vi "Save_Ensight.vi"() -> (5 "Plug in titles":string[](array[string]), 7 "Plug in values":string[](array[string]))   [LabVIEW 2011]
uses:
  Globals/Plug_in_data_global.vi
  Globals/LDA_meas_global_1.vi
  Globals/Meas_global.vi
  Globals/Constants_global.vi
  <vilib>/ptbypt/NI_PtbyPt.lvlib
panel:
  out "Temp File Path":path
  out "concatenated string":string
  out "Results Array":string[](array[string])
  out "IJ Values":i32[](array[numeric])
  out "Latest Data":dbl[][](array[numeric])
  out "Variables":dbl[][](array[numeric])
  out "Results File Path":path
  out "Processing first block?":bool
  out "XY Position":string[](array[string])
  out "Results File Exists?":bool
  # "You must have just these two indicators on the connector pane of the vi"
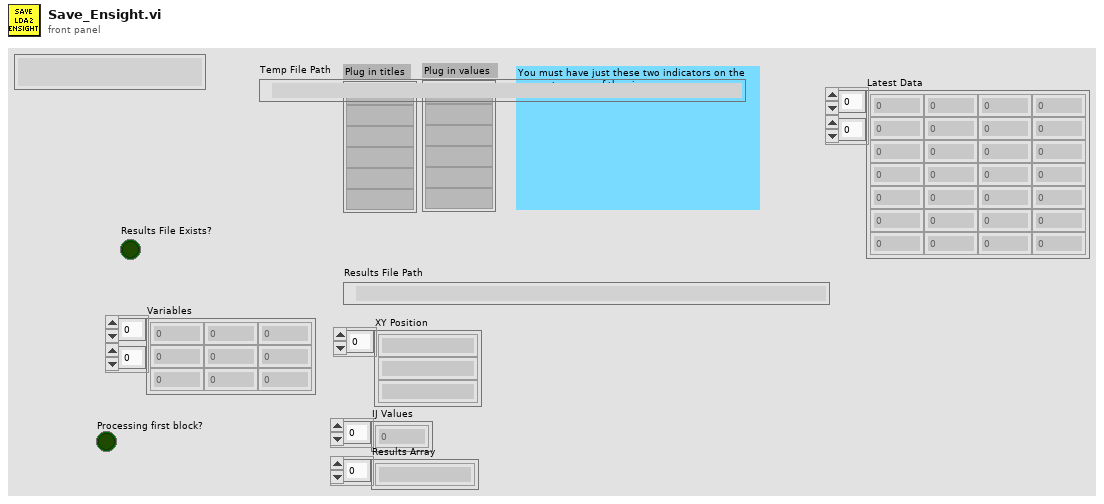
[diagram p1: front panel]
types:
  T1 = typedef "Analysis_info_cluster.ctl" = cluster{"Colour":u32, "Inst type":T2, "Inst name":string, "Symbol":string, "Code name":string, "Extra Info":string, "Inst Array":T3, "Index":i32, "Voltage Index":i32, "Extra Titles":string[], "Extra Values":string[], "Eng Values":dbl[], "Time (ms)":dbl[], "Voltage":dbl[], "U":dbl, "u^2":dbl, "u^3":dbl, "u^4":dbl, "Skew_u":dbl, "Kurt_u":dbl, "Sd Error in Mean":dbl, "% u'/U":dbl, "X":dbl, "Y":dbl, "Z":dbl, "Spectra":T4, "Autocorrelation":T4, "Timescale integral to 25%":dbl, "Sd Error in Variance":dbl, "Calib File":path, "Calib Constants":dbl[], "Histogram":T4, "Output Position":bool, "Full Stats":bool, "Weighting":dbl[]}
  T2 = typedef "Inst_type.ctl" = enum16{"Propeller anemometer", "Raw voltage", "Pressure Transducer", "Pitot-static tube", "Preston tube", "Hot wire", "Cross wire 1", "Cross wire 2", "Generic Linear", "Generic Polynomial", "Generic BackPoly", "Fast FID", "Thermocouple", "Cold wire", "Pulsed Wire", "LDA Vel", "LDA Tran time", "LDA Arr time"}
  T3 = typedef "Instrument_Array.ctl" = enum16{"PWA", "LDA", "Analogue"}
  T4 = typedef "XY_Plot_Cluster.ctl" = cluster{"First Name":string, "Second Name":string, "X axis name":string, "Y axis name":string, "X array":dbl[], "Y array":dbl[]}
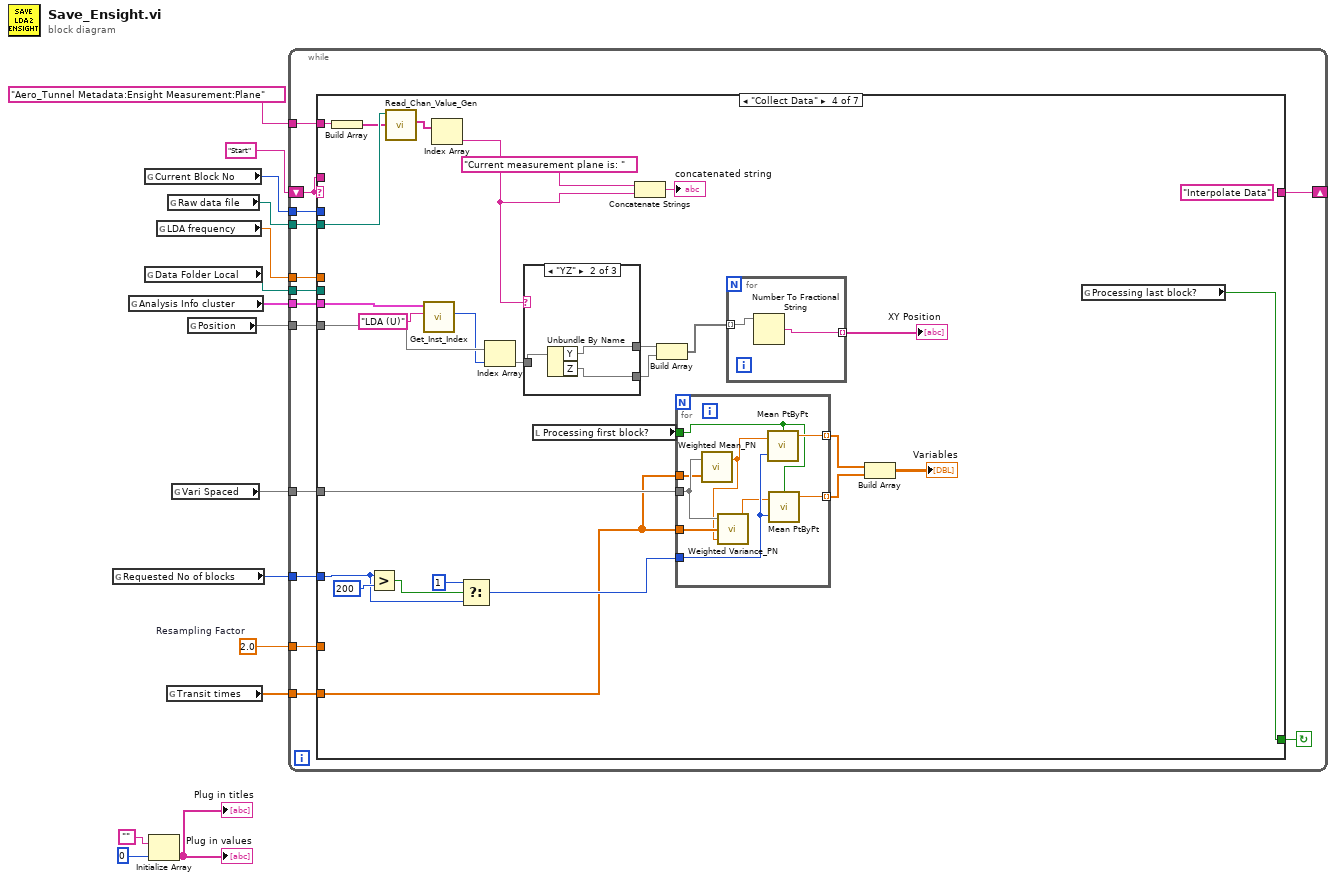
[diagram p0: block diagram]
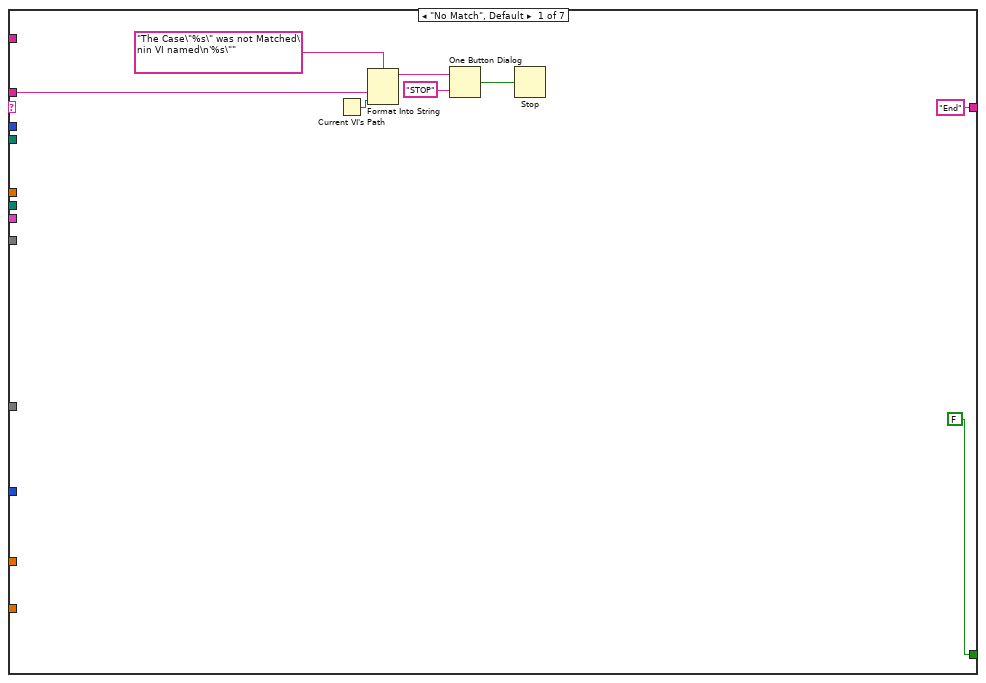
[diagram p2: hidden frame]
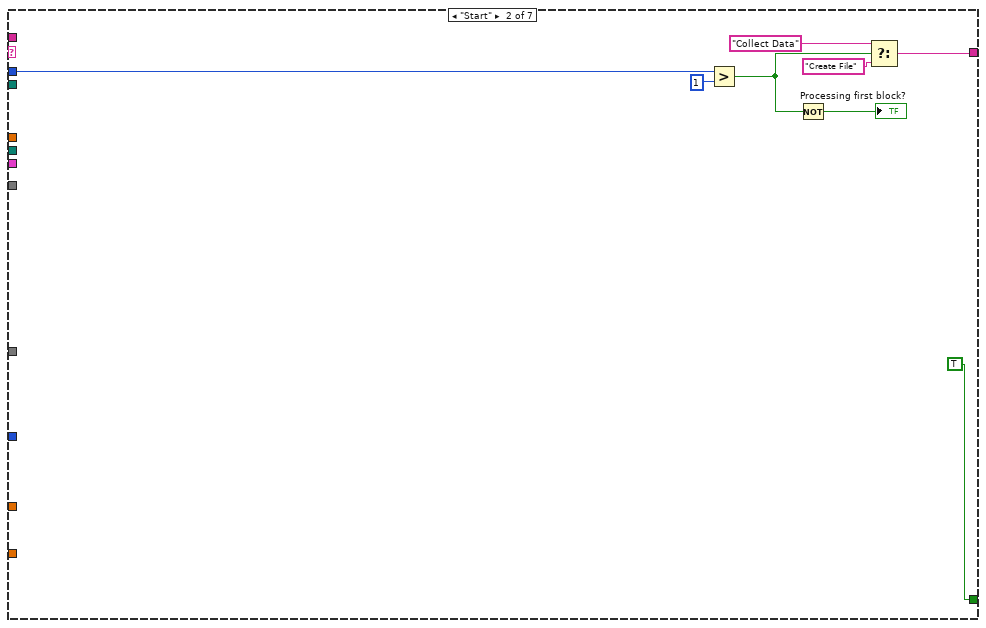
[diagram p3: hidden frame]
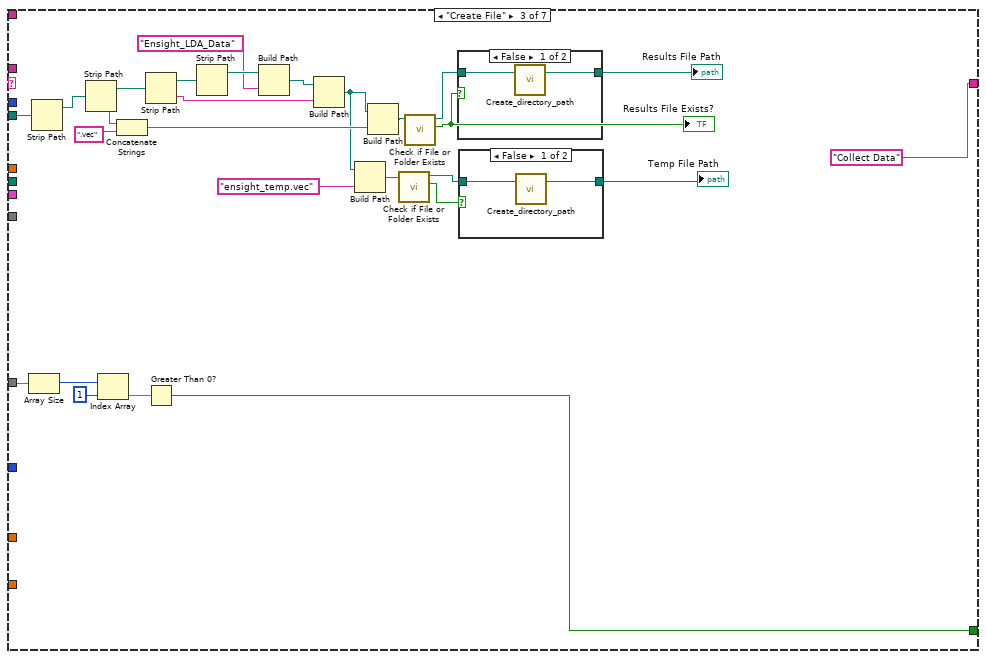
[diagram p4: hidden frame]
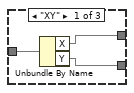
[diagram p7: hidden frame]
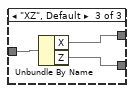
[diagram p8: hidden frame]
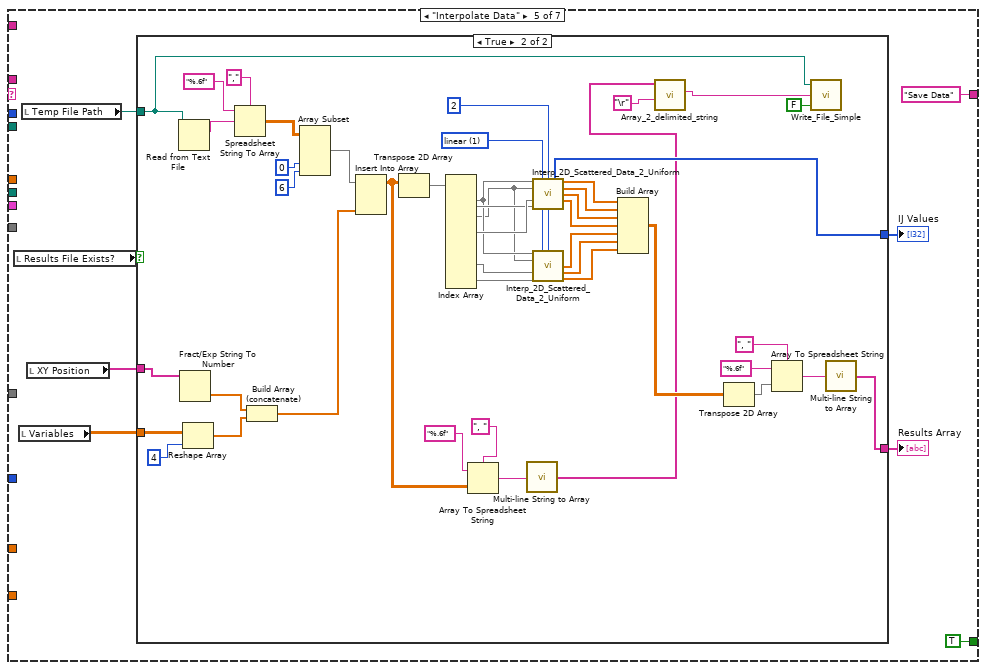
[diagram p9: hidden frame]
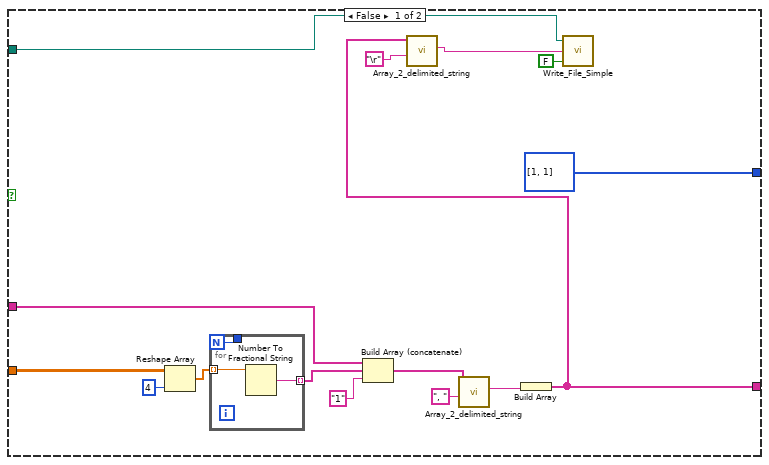
[diagram p10: hidden frame]
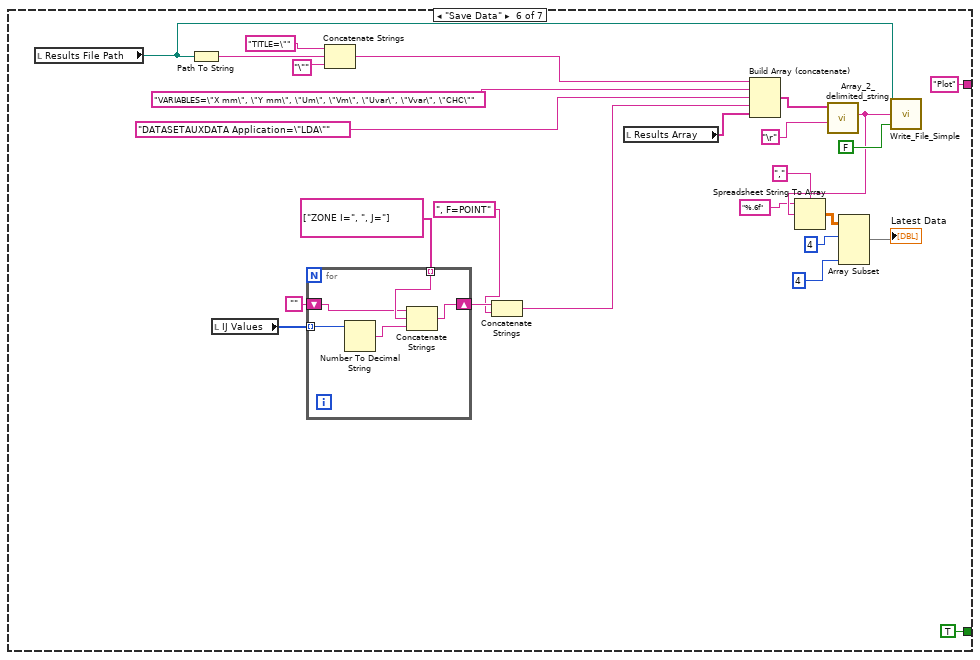
[diagram p11: hidden frame]
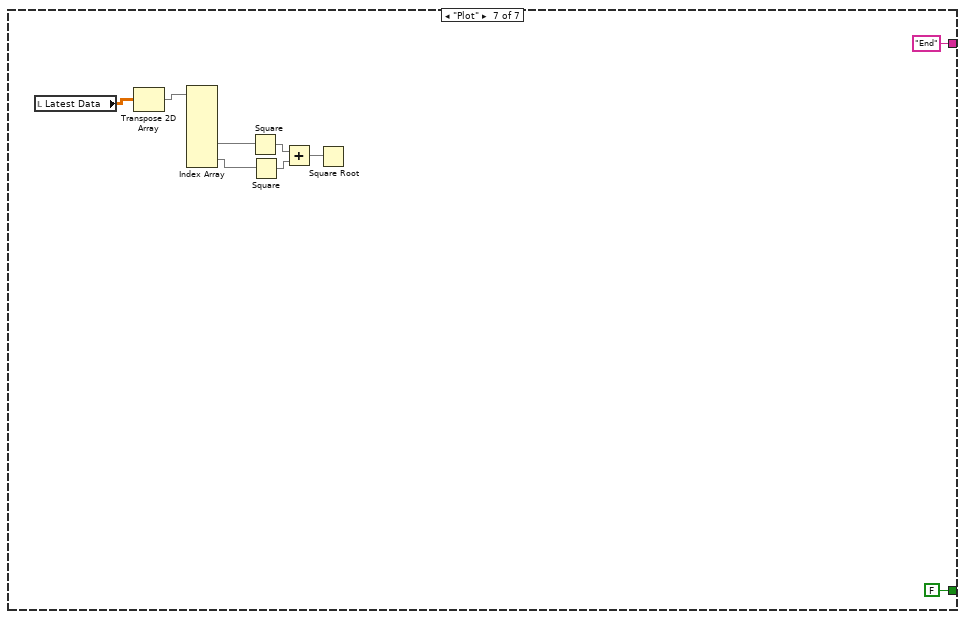
[diagram p12: hidden frame]
diagram:
  w6 = 2.0  # Resampling Factor
  n1 = global read "Meas_global.vi" "Requested No of blocks"() -> (w3:i32)
  n2 = global read "Meas_global.vi" "Analysis Info cluster"() -> (w4:T1[])
  n3 = global read "Meas_global.vi" "Current Block No"() -> (w9:i32)
  n4 = global read "Constants_global.vi" "Data Folder Local"() -> (w5:path)
  n5 = Initialize Array("", 0) -> (→"Plug in values" →"Plug in titles":string[])
  n6 = global read "Meas_global.vi" "LDA frequency"() -> (w7:dbl)
  n7 = global read "LDA_meas_global_1.vi" "Transit times"() -> (w13:dbl[])
  n8 = global read "Meas_global.vi" "Raw data file"() -> (w8:path)
  n9 = global read "Plug_in_data_global.vi" "Vari Spaced"() -> (w14)
  n10 = global read "Meas_global.vi" "Position"() -> (w2)
  n11 = while {
    shift-left: "Start" -> [w29]
    shift-right: [w26] -> _
    tunnel: w14 -> [w28]
    tunnel: w13 -> [w27]
    tunnel: w9 -> [w24]
    tunnel: w5 -> [w23]
    tunnel: w8 -> [w22]
    tunnel: w7 -> [w21]
    tunnel: w6 -> [w20]
    tunnel: w4 -> [w19]
    tunnel: w3 -> [w18]
    tunnel: w2 -> [w17]
    tunnel: "Aero_Tunnel Metadata:Ensight Measurement:Plane" -> [w16]
    stop <- w25 continue-if-true
    n12 = case shown="\"Collect Data\"" w29 {
      tunnel: ["End" ("t") w40 "Collect Data" ("t") "Interpolate Data" ("t") "Save Data" ("t") "Plot" ("t") "End" ("t")] -> w26
      tunnel: w29 -> [w33 _ _ _ _ _ _]
      tunnel: w28 -> [_ _ w71 w106 _ _ _]
      tunnel: w27 -> [_ _ _ w99 _ _ _]
      tunnel: [FALSE TRUE w67 w86 TRUE ("Processing last block?") TRUE ("Processing last block?") FALSE ("Processing last block?")] -> w25
      tunnel: w24 -> [_ w39 _ _ _ _ _]
      tunnel: w23 -> [_ _ _ _ _ _ _]
      tunnel: w22 -> [_ _ w66 w85 _ _ _]
      tunnel: w21 -> [_ _ _ _ _ _ _]
      tunnel: w20 -> [_ _ _ _ _ _ _]
      tunnel: w19 -> [_ _ _ w96 _ _ _]
      tunnel: w18 -> [_ _ _ w101 _ _ _]
      tunnel: w17 -> [_ _ _ w98 _ _ _]
      tunnel: w16 -> [_ _ _ w84 _ _ _]
      frame "No Match", Default {
        n13 = Current VI's Path() -> (path=w32:path)
        n14 = Format Into String(format string="The Case\"%s\" was not Matched\nin VI named\n'%s\"" ("Format String"), w33, w32) -> (resulting string=w36:string)  [unwired: 2 in, 1 out]
        n15 = One Button Dialog(message=w36, button name ("OK")="STOP") -> (true=w34:bool)
        n16 = Stop(stop? (T)=w34) -> ()
      }
      frame "Start" {
        n17 = Greater?(x=w39, y=1) -> (0:w42:bool)
        n18 = Not(x=w42) -> (.not. x?=→"Processing first block?":bool)
        n19 = Select(t="Collect Data", s=w42, f="Create File") -> (s? t:f=w40:string)
      }
      frame "Create File" {
        n20 = Array Size(array=w71) -> (size(s)=w70:i32)
        n21 = Strip Path(path=w66) -> (stripped path=w65:path)  [unwired: 1 out]
        n22 = Strip Path(path=w65) -> (stripped path=w64:path, name=w53:string)
        n23 = Index Array(array=w70, index=1) -> (element=w68)
        n24 = Concatenate Strings(w53, ".vec" ("string")) -> (w57:string)
        n25 = Strip Path(path=w64) -> (stripped path=w63:path, name=w59:string)
        n26 = Greater Than 0?(x=w68) -> (x > 0?=w67:bool)
        n27 = Strip Path(path=w63) -> (stripped path=w62:path)  [unwired: 1 out]
        n28 = Build Path(base path=w62, name or relative path="Ensight_LDA_Data") -> (appended path=w60:path)
        n29 = Build Path(base path=w60, name or relative path=w59) -> (appended path=w49:path)
        n30 = Build Path(base path=w49, name or relative path="ensight_temp.vec" ("string")) -> (appended path=w51:path)
        n31 = Build Path(base path=w49, name or relative path=w57) -> (appended path=w52:path)
        n32 = call <vilib>:"Check if File or Folder Exists.vi"("path"=w51) -> ("file or folder exists?"=w48:bool, "dup path"=w47:path)  [unwired: 8 in, 1 out]
        n33 = call <vilib>:"Check if File or Folder Exists.vi"("path"=w52) -> ("file or folder exists?"=w54:bool, "dup path"=w56:path)  [unwired: 8 in, 1 out]
        "Results File Exists?" <- w54
        n34 = case shown="False" w54 {
          tunnel: w56 -> [w77 w78]
          tunnel: [w76 w78] -> w55
          frame False {
            n35 = call "Create_directory_path.vi"("Path name"=w77) -> ("Path name Out"=w76:path)  [unwired: 1 in, 1 out]
          }
          frame True {
          }
        }
        "Results File Path" <- w55
        n36 = case shown="False" w48 {
          tunnel: w47 -> [w74 w75]
          tunnel: [w73 w75] -> w46
          frame False {
            n37 = call "Create_directory_path.vi"("Path name"=w74) -> ("Path name Out"=w73:path)  [unwired: 1 in, 1 out]
          }
          frame True {
          }
        }
        "Temp File Path" <- w46
      }
      frame "Collect Data" {
        n38 = Build Array(w84) -> (w83:string[])
        n39 = Greater?(x=w101, y=200) -> (0:w103:bool)
        n40 = call "Read_Chan_Value_Gen.vi"("Desired Ch Names"=w83, "Raw data file"=w85) -> ("Values"=w82:string[])  [unwired: 9 in]
        n41 = call "Get_Inst_Index.vi"("Inst name search"="LDA (U)", 11:w96) -> ("Index of Instance"=w95:i32)  [unwired: 7 in, 2 out]
        n42 = Index Array(array=w82) -> (element=w81:string)  [unwired: 1 in]
        n43 = Select(t=1, s=w103, f=w101) -> (s? t:f=w100:i32)
        n44 = Index Array(array=w98, index=w95) -> (element=w94)
        n45 = case shown="\"YZ\"" w81 {
          tunnel: w94 -> [w110 w113 w116]
          tunnel: [w109 w112 w115] -> w93
          tunnel: [w108 w111 w114] -> w92
          frame "XY" {
            n46 = Unbundle By Name(w110) -> ("X"=w109, "Y"=w108)
          }
          frame "YZ" {
            n47 = Unbundle By Name(w113) -> ("Y"=w112, "Z"=w111)
          }
          frame "XZ", Default {
            n48 = Unbundle By Name(w116) -> ("X"=w115, "Z"=w114)
          }
        }
        n49 = local read "Processing first block?"() -> (w105:bool)
        n50 = Concatenate Strings("Current measurement plane is: " ("string"), w81) -> (→"concatenated string":string)
        n51 = Build Array(w93, w92) -> (w88:void[])
        n52 = for {
          tunnel: w106 -> [w123]
          tunnel: [w127] -> w91 mode=indexing
          tunnel: [w126] -> w90 mode=indexing
          tunnel: w105 -> [w124]
          tunnel: w100 -> [w125]
          tunnel: w99 -> [w122]
          tunnel: w99 -> [w121]
          n53 = call "Weighted Mean_PN.vi"("weights"=w121, "1D data"=w123) -> ("Weighted mean"=w120:dbl)  [unwired: 1 in]
          n54 = call "Weighted Variance_PN.vi"("Weighted mean"=w120, "weights"=w122, "1D data"=w123) -> ("Weighted variance"=w119:dbl)  [unwired: 1 in]
          n55 = call <vilib>:"Mean PtByPt.vi"("x"=w120, "sample length"=w125, "initialize"=w124) -> ("mean"=w127:dbl)  [unwired: 1 in, 1 out]
          n56 = call <vilib>:"Mean PtByPt.vi"("x"=w119, "sample length"=w125, "initialize"=w124) -> ("mean"=w126:dbl)  [unwired: 1 in, 1 out]
        }
        n57 = for {
          tunnel: w88 -> [w118] mode=indexing
          tunnel: [w117] -> w87 mode=indexing
          n58 = Number To Fractional String(number=w118) -> (F-format string=w117:string)  [unwired: 3 in]
        }
        "XY Position" <- w87
        n59 = Build Array(w91, w90) -> (→"Variables":dbl[][])
        n60 = global read "Meas_global.vi" "Processing last block?"() -> (w86:bool)
      }
      frame "Interpolate Data" {
        n61 = local read "Results File Exists?"() -> (w131:bool)
        n62 = local read "Variables"() -> (w133:dbl[][])
        n63 = local read "Temp File Path"() -> (w128:path)
        n64 = local read "XY Position"() -> (w132:string[])
        n65 = case shown="True" w131 {
          tunnel: w133 -> [w150 w191]
          tunnel: [w139 w166] -> w129
          tunnel: w132 -> [w144 w192]
          tunnel: [i32[] [1, 1] w179] -> w130
          tunnel: w128 -> [w136 w162]
          frame False {
            n66 = Reshape Array(w150, 4 ("dimension size")) -> (w148:dbl[])
            n67 = for {
              N -> [w151]
              tunnel: w148 -> [w153] mode=indexing
              tunnel: [w152] -> w145 mode=indexing
              tunnel: [w151] -> _
              n68 = Number To Fractional String(number=w153) -> (F-format string=w152:string)  [unwired: 3 in]
            }
            n69 = Build Array (concatenate)(w144, w145, "1") -> (w143:string[])
            n70 = call "Array_2_delimited_string.vi"("delimiter (Tab)"=", ", "Array of Strings"=w143) -> ("delimited string"=w146:string)  [unwired: 9 in]
            n71 = Build Array(w146) -> (w139:string[])
            n72 = call "Array_2_delimited_string.vi"("delimiter (Tab)"="\r", "Array of Strings"=w139) -> ("delimited string"=w138:string)  [unwired: 9 in]
            n73 = call "Write_File_Simple.vi"("append to file? (new file:F)"=FALSE, "character string"=w138, "file path"=w136) -> ()  [unwired: 2 out]
          }
          frame True {
            w177 = 2 ("Interpolation Factor")
            w178 = 1 items=["nearest", "linear", "cubic", "biharmonic spline "] ("method")
            n74 = Read from Text File(file (use dialog)=w162) -> (text=w194:string)  [unwired: 3 in, 3 out]
            n75 = Fract/Exp String To Number(string=w192) -> (number=w189:dbl[])  [unwired: 3 in, 1 out]
            n76 = Reshape Array(w191, 4 ("index")) -> (w188:dbl[])
            n77 = Spreadsheet String To Array(delimiter (Tab)=",", format string="%.6f", spreadsheet string=w194) -> (array=w193:dbl[][])  [unwired: 1 in]
            n78 = Build Array (concatenate)(w189, w188) -> (w186:dbl[])
            n79 = Array Subset(array=w193, index (col)=0 ("index"), length (col)=6 ("length")) -> (w187:dbl[][])  [unwired: 2 in]
            n80 = Insert Into Array(array=w187, new element=w186) -> (w156:dbl[][])  [unwired: 2 in]
            n81 = Transpose 2D Array(2D array=w156) -> (transposed array=w185:dbl[][])
            n82 = Index Array(array=w185) -> (element #1=w182:dbl[], element #2=w154:dbl[], element #3=w184:dbl[], element #4=w183:dbl[], element #5=w181:dbl[], element #6=w180:dbl[])  [unwired: 12 in]
            n83 = Array To Spreadsheet String(delimiter (Tab)=", ", array=w156, 3:"%.6f" ("format string")) -> (spreadsheet string=w161:string)
            n84 = call "Multi-line String to Array.vi"("Multi lined string"=w161) -> ("Array of string lines"=w155:string[])
            n85 = call "Interp_2D_Scattered_Data_2_Uniform.vi"("X"=w182, "method"=w178, "Interpolation Factor"=w177, "Y"=w154, "U"=w184, "V"=w183) -> ("IJ Values"=w179:i32[], "Xi"=w176:dbl[], "Yi"=w175:dbl[], "Ui"=w174:dbl[], "Vi"=w173:dbl[])  [unwired: 4 in, 1 out]
            n86 = call "Interp_2D_Scattered_Data_2_Uniform.vi"("X"=w182, "method"=w178, "Interpolation Factor"=w177, "Y"=w154, "U"=w181, "V"=w180) -> ("Ui"=w172:dbl[], "Vi"=w171:dbl[], "Convex Hull Check"=w170:dbl[])  [unwired: 4 in, 3 out]
            n87 = Build Array(w176, w175, w174, w173, w172, w171, w170) -> (w168:dbl[][])
            n88 = call "Array_2_delimited_string.vi"("delimiter (Tab)"="\r", "Array of Strings"=w155) -> ("delimited string"=w164:string)  [unwired: 9 in]
            n89 = Transpose 2D Array(2D array=w168) -> (transposed array=w169:dbl[][])
            n90 = Array To Spreadsheet String(delimiter (Tab)=", ", array=w169, 3:"%.6f" ("format string")) -> (spreadsheet string=w167:string)
            n91 = call "Write_File_Simple.vi"("append to file? (new file:F)"=FALSE, "character string"=w164, "file path"=w162) -> ()  [unwired: 2 out]
            n92 = call "Multi-line String to Array.vi"("Multi lined string"=w167) -> ("Array of string lines"=w166:string[])
          }
        }
        "IJ Values" <- w130
        "Results Array" <- w129
      }
      frame "Save Data" {
        n93 = local read "Results File Path"() -> (w208:path)
        n94 = Path To String(path=w208) -> (string=w221:string)
        n95 = local read "IJ Values"() -> (w201:i32[])
        n96 = for {
          tunnel: w201 -> [w229] mode=indexing
          shift-right: [w227] -> w204
          shift-left: "" -> [w225]
          tunnel: string[] ["ZONE I=", ", J="] -> [w226] mode=indexing
          n97 = Number To Decimal String(number=w229) -> (decimal integer string=w228:string)  [unwired: 1 in]
          n98 = Concatenate Strings(w225, w226, w228) -> (w227:string)
        }
        n99 = Concatenate Strings("TITLE=\"" ("string"), w221, "\"" ("string")) -> (w219:string)
        n100 = Concatenate Strings(w204, ", F=POINT") -> (w202:string)
        n101 = local read "Results Array"() -> (w200:string[])
        n102 = Build Array (concatenate)(w219, "VARIABLES=\"X mm\", \"Y mm\", \"Um\", \"Vm\", \"Uvar\", \"Vvar\", \"CHC\"" ("string"), "DATASETAUXDATA Application=\"LDA\"", w202, w200) -> (w216:string[])
        n103 = call "Array_2_delimited_string.vi"("delimiter (Tab)"="\r", "Array of Strings"=w216) -> ("delimited string"=w214:string)  [unwired: 9 in]
        n104 = Spreadsheet String To Array(delimiter (Tab)=",", format string="%.6f", spreadsheet string=w214) -> (array=w213:dbl[][])  [unwired: 1 in]
        n105 = Array Subset(array=w213, index (row)=4 ("index"), length (col)=4 ("length")) -> (→"Latest Data":dbl[][])  [unwired: 2 in]
        n106 = call "Write_File_Simple.vi"("append to file? (new file:F)"=FALSE, "character string"=w214, "file path"=w208) -> ()  [unwired: 2 out]
      }
      frame "Plot" {
        n107 = local read "Latest Data"() -> (w236:dbl[][])
        n108 = Transpose 2D Array(2D array=w236) -> (transposed array=w235:dbl[][])
        n109 = Index Array(array=w235) -> (element #3=w234:dbl[], element #4=w233:dbl[])  [unwired: 8 in, 2 out]
        n110 = Square(x=w234) -> (x^2=w232:dbl[])
        n111 = Square(x=w233) -> (x^2=w231:dbl[])
        n112 = Add(x=w232, y=w231) -> (x+y=w230:dbl[])
        n113 = Square Root(x=w230) -> ()  [unwired: 1 out]
      }
    }
  }
